vi "Close FPGA.vi"(8 "error in (no error)":errorcluster, 11 "Generic FPGA Reference":T1) -> (0 "error out":errorcluster)   [LabVIEW 2013, in "SGDV_Ctrl_v13_lib.lvlib"]
uses:
  SGDV_Ctrl_v13_lib.lvlib
  <vilib>/myRIO/Common/Instrument Driver Framework/Utilities/typedefs/Generic FPGA Reference.ctl
  <vilib>/myRIO/Common/Instrument Driver Framework/myRIO v1.0/UART/vis/myRIO v1.0 Close UART.vi
  <vilib>/myRIO/Common/Instrument Driver Framework/Utilities/vis/FPGA Ref Manager.vi
  <vilib>/myRIO/Common/Instrument Driver Framework/myRIO v1.0/myRIO v1.0 Reset FPGA.vi
  <vilib>/FPGAPlugInAG/Dynamic/niLvFpga_Abort_Dynamic.vi
  <vilib>/FPGAPlugInAG/Dynamic/niLvFpga_Close_Dynamic.vi
  <vilib>/rvi/interface/nirviMethod/nirviMethod.xnode
  <vilib>/rvi/interface/nirviCloseFPGA/nirviCloseFPGA.xnode
  <vilib>/myRIO/Instrument Drivers/Utilities/Utilities.lvlib
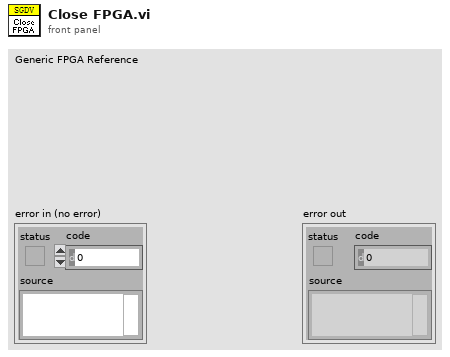
[diagram p1: front panel]
types:
  T1 = typedef "Generic FPGA Reference.ctl" = refnum<k20>
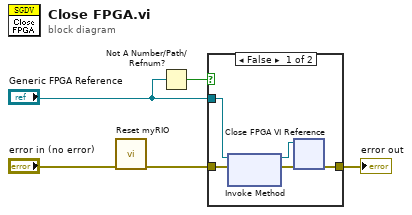
[diagram p0: block diagram]
diagram:
  n1 = call <vilib>:"Reset myRIO.vi"("error in (no error)"="error in (no error)") -> ("error out"=w4:errorcluster)  [unwired: 10 in]
  n2 = Not A Number/Path/Refnum?(number/path/refnum="Generic FPGA Reference") -> (NaN/Path/Refnum?=w5:bool)
  n3 = case shown="False" w5 {
    tunnel: "Generic FPGA Reference" -> [w10 _]
    tunnel: [w7 w11] -> w2
    tunnel: w4 -> [w6 w11]
    frame False {
      n4 = xnode "Invoke Method"("FPGA VI Reference In"=w10, "error in"=w6) -> ("FPGA VI Reference Out"=w9:T1, "error out"=w8:errorcluster)
      n5 = xnode "Close FPGA VI Reference"("FPGA VI Reference In"=w9, "error in"=w8) -> ("error out"=w7:errorcluster)
    }
    frame True {
    }
  }
  "error out" <- w2
